vi "UIRefs Full Scale Range.vi"(8 "error in (no error)":errorcluster, 11 "FC2901 in":refnum<class "FC2901.lvclass">) -> (0 "error out":errorcluster, 3 "FC2901 out":refnum<class "FC2901.lvclass">)   [LabVIEW 2021, in "FC2901.lvclass"]
uses:
  FC2901.lvclass
  FC2901.lvclass/FC2901.ctl
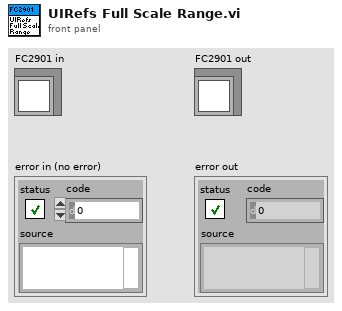
[diagram p1: front panel]
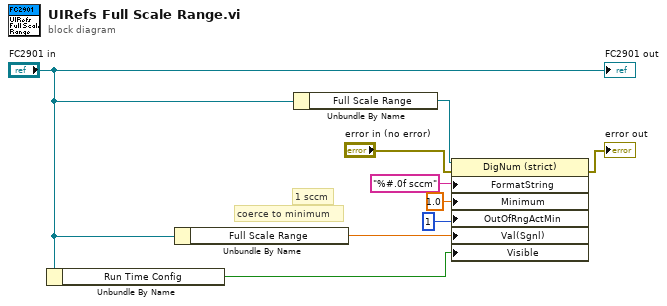
[diagram p0: block diagram]
diagram:
  # "coerce to minimum"
  # "1 sccm"
  n1 = Unbundle By Name("FC2901 in") -> ("Run Time Config"=w3:bool)
  n2 = Unbundle By Name("FC2901 in") -> ("Full Scale Range"=w5:dbl)
  n3 = Unbundle By Name("FC2901 in") -> ("Full Scale Range"=w9:refnum<vi>)
  n4 = property class="DigNum (strict)"(reference=w9, error in="error in (no error)", "FormatString"="%#.0f sccm" ("Format String"), "Minimum"=1.0 ("Data Entry Limits:Minimum"), "OutOfRngActMin"=u8 1 ("Response to Value Outside Limits:Minimum"), "Val(Sgnl)"=w5, "Visible"=w3) -> (error out=→"error out":errorcluster)  [unwired: 1 out]
  "FC2901 out" <- "FC2901 in"
